vi "StepToMTRTEQC.vi"(10 "StationIn":string) -> (2 "StationOut":string)   [LabVIEW 2012]
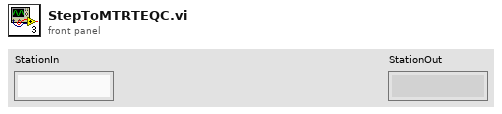
[diagram p1: front panel]
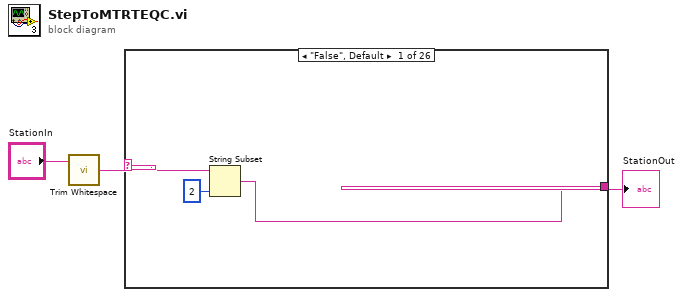
[diagram p0: block diagram]
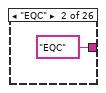
[diagram p2: hidden frame]
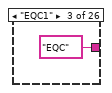
[diagram p3: hidden frame]
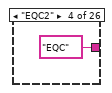
[diagram p4: hidden frame]
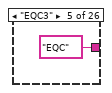
[diagram p5: hidden frame]
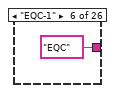
[diagram p6: hidden frame]
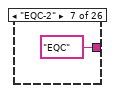
[diagram p7: hidden frame]
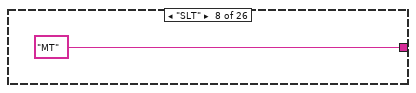
[diagram p8: hidden frame]
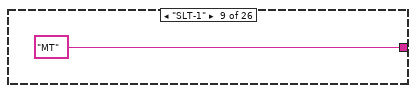
[diagram p9: hidden frame]
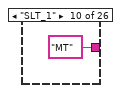
[diagram p10: hidden frame]
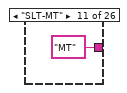
[diagram p11: hidden frame]
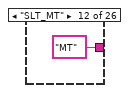
[diagram p12: hidden frame]
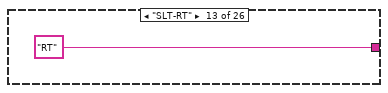
[diagram p13: hidden frame]
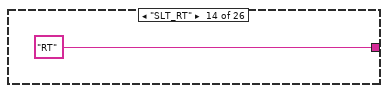
[diagram p14: hidden frame]
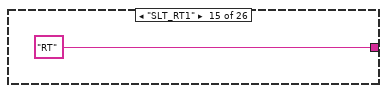
[diagram p15: hidden frame]
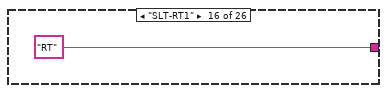
[diagram p16: hidden frame]
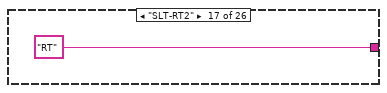
[diagram p17: hidden frame]
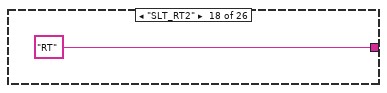
[diagram p18: hidden frame]
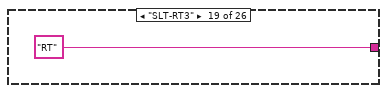
[diagram p19: hidden frame]
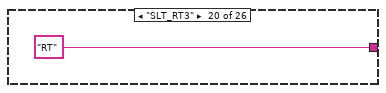
[diagram p20: hidden frame]
diagram:
  n1 = call <vilib>:"Trim Whitespace.vi"("string"="StationIn") -> ("trimmed string"=w2:string)  [unwired: 1 in]
  n2 = case shown="\"False\", Default" w2 {
    selector: w2 -> [w5 _ _ _ _ _ _ _ _ _ _ _ _ _ _ _ _ _ _ _ _ _ _ _ _ _]
    tunnel: [w4 "EQC" "EQC" "EQC" "EQC" "EQC" "EQC" "MT" "MT" "MT" "MT" "MT" "RT" "RT" "RT" "RT" "RT" "RT" "RT" "RT" "RT" "RT" "EQC" "EQC" "ENG" "ENG"] -> w1
    frame "False", Default {
      n3 = String Subset(string=w5, length (rest)=2 ("length (rest)")) -> (substring=w4:string)  [unwired: 1 in]
    }
    frame "EQC" {
    }
    frame "EQC1" {
    }
    frame "EQC2" {
    }
    frame "EQC3" {
    }
    frame "EQC-1" {
    }
    frame "EQC-2" {
    }
    frame "SLT" {
    }
    frame "SLT-1" {
    }
    frame "SLT_1" {
    }
    frame "SLT-MT" {
    }
    frame "SLT_MT" {
    }
    frame "SLT-RT" {
    }
    frame "SLT_RT" {
    }
    frame "SLT_RT1" {
    }
    frame "SLT-RT1" {
    }
    frame "SLT-RT2" {
    }
    frame "SLT_RT2" {
    }
    frame "SLT-RT3" {
    }
    frame "SLT_RT3" {
    }
    frame "SLT-RT4" {
    }
    frame "SLT_RT4" {
    }
    frame "SLT-EQC" {
    }
    frame "SLT_EQC" {
    }
    frame "TEST" {
    }
    frame "TEST-FAIL" {
    }
  }
  "StationOut" <- w1
